vi "Global GPS.vi"() -> ()   [LabVIEW 2014]
panel:
  in  "output cluster":T1
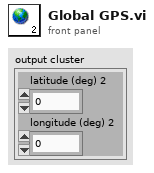
[diagram p1: front panel]
types:
  T1 = cluster{"latitude (deg) 2":dbl, "longitude (deg) 2":dbl}
diagram:
